vi "Split String Array By Patterns_CSM.vi"(8 "Patterns":string[](array[string]), 11 "Text Array":string[](array[string])) -> (3 "Array":cluster{"filtered array":string[]}[](array[cluster]))   [LabVIEW 2017, in "csm-file-support.lvlib"]
uses:
  csm-file-support.lvlib
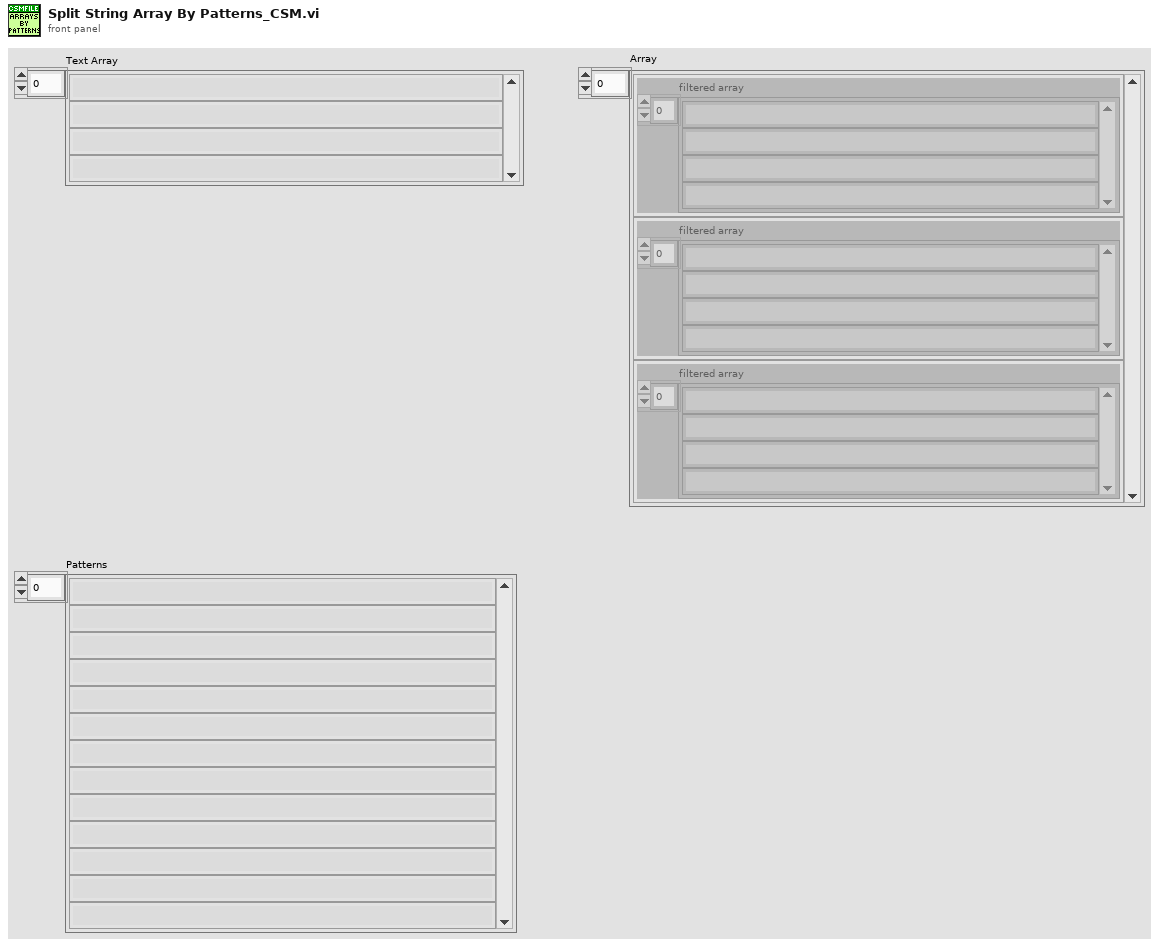
[diagram p1: front panel]
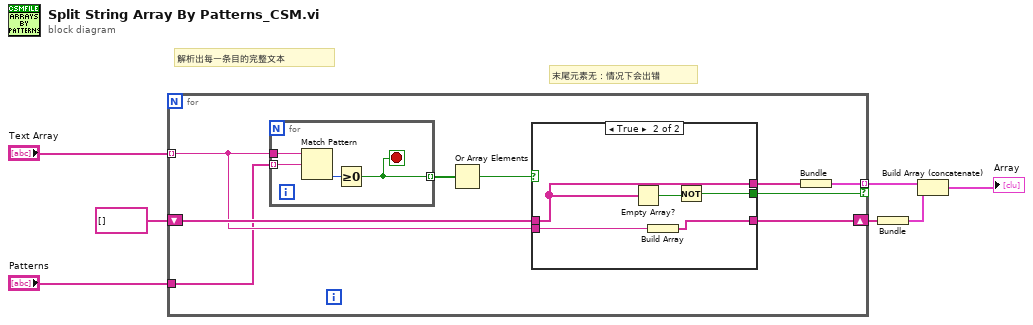
[diagram p0: block diagram]
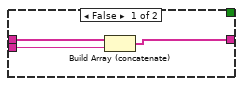
[diagram p2: hidden frame]
diagram:
  # "解析出每一条目的完整文本"
  # "末尾元素无：情况下会出错"
  n1 = for {
    tunnel: "Text Array" -> [w15] mode=indexing
    shift-right: [w14] -> w5
    shift-left: string[] [] -> [w16]
    tunnel: [w11] -> w7 mode=indexing if=w10
    tunnel: "Patterns" -> [w9]
    n2 = for {
      tunnel: w15 -> [w19]
      tunnel: [w17] -> w12 mode=indexing
      tunnel: w9 -> [w18] mode=indexing
      stop <- w17 stop-if-true
      n3 = Match Pattern(string=w19, regular expression=w18) -> (offset past match=w20:i32)  [unwired: 1 in, 3 out]
      n4 = Greater Or Equal To 0?(x=w20) -> (x >= 0?=w17:bool)
    }
    n5 = Or Array Elements(Boolean array=w12) -> (logical OR=w8:bool)
    n6 = case shown="True" w8 {
      tunnel: w16 -> [w23 w24]
      tunnel: w15 -> [w22 w28]
      tunnel: [w21 w27] -> w14
      tunnel: [_ w24] -> w13
      tunnel: [_ w25] -> w10
      frame False {
        n7 = Build Array (concatenate)(w23, w22) -> (w21:string[])
      }
      frame True {
        n8 = Empty Array?(array=w24) -> (empty?=w26:bool)
        n9 = Build Array(w28) -> (w27:string[])
        n10 = Not(x=w26) -> (.not. x?=w25:bool)
      }
    }
    n11 = Bundle(w13) -> (w11:cluster{string[]})  [unwired: 1 in]
  }
  n12 = Bundle(w5) -> (w4:cluster{string[]})  [unwired: 1 in]
  n13 = Build Array (concatenate)(w7, w4) -> (→"Array":cluster{string[]}[])
